vi "CCD.vi"() -> ()   [LabVIEW 2016]
uses:
  <vilib>/userdefined/High Color/IMAQdx.ctl
  <vilib>/UPVI/lvhdf5/file.llb/LVH5F Operation.ctl
  <vilib>/UPVI/lvhdf5/dataset.llb/LVH5D Operation.ctl
  <vilib>/Utility/miscctls.llb/LVRectTypeDef.ctl
  <vilib>/UPVI/lvhdf5/group.llb/H5G_obj_t.ctl
  <vilib>/UPVI/lvhdf5/utility.llb/Select HDF5 Dialog.vi
  <vilib>/UPVI/lvhdf5/utility.llb/Select HDF5 Dialog (Object Only).vi
  <vilib>/UPVI/lvhdf5/dataset.llb/Simple H5Dwrite (Variant).vi
  <vilib>/UPVI/lvhdf5/dataset.llb/Simple H5Dwrite.xnode
  <vilib>/UPVI/lvhdf5/library.llb/HDF5 Ref.ctl
  <vilib>/vision/driver/NI_Vision_Acquisition_Software.lvlib
  <instrlib>/Ocean Optics 2000 4000/Ocean Optics 2000 4000.lvlib
  <vilib>/UPVI/lvhdf5/identifier.llb/Not an HDF5 Refnum Constant.vi
  <vilib>/Utility/error.llb/Error Cluster From Error Code.vi
  <vilib>/UPVI/lvhdf5/dataset.llb/OpenCreateReplace Dataset by Element Type.vi
  <vilib>/UPVI/lvhdf5/dataspace.llb/H5Sselect_hyperslab.vi
  <vilib>/UPVI/lvhdf5/dataset.llb/H5Dwrite (Variant).vi
  <vilib>/UPVI/lvhdf5/dataset.llb/H5Dget_space.vi
  <vilib>/UPVI/lvhdf5/attribute.llb/private/LVH5AwriteWDTAttrs.vi
  <vilib>/UPVI/lvhdf5/dataspace.llb/H5Sclose.vi
  <vilib>/UPVI/lvhdf5/dataset.llb/H5Dclose.vi
  <vilib>/UPVI/lvhdf5/utility.llb/Select HDF5 Dialog (File and Object).vi
panel:
  in  "Tiempo entre muestra (ms)":u32=1000
  in  "Guarda":bool
  out "vy":dbl(slide) scale=-10.0..10.0
  in  "Tiempo de avanze (ms)":u32=100
  in  "Valor final en y":dbl
  in  "Movimiento de spot en y":dbl(slide) scale=-10.0..10.0
  in  "Valor final en  x":dbl
  in  "Paso":dbl=0.01
  out "vx":dbl(slide) scale=-10.0..10.0
  in  "Modo de operación":enum32{"Manual", "Mapeo"}(radio)
  in  "stop":bool
  in  "Movimiento de spot en x":ext(slide) scale=-10.0..10.0
  in  "error in":errorcluster
  out "Guarda datos":bool
  in  "Ruta":path=path "C:/Users/Posgrado/Desktop/Test/Prueba"
  in  "Dataset Path":string="Mapeo"
  in  "No. de muestras":i32=1
  in  "Session In":T1="cam2"
  in  "Enable Strobe (Disabled)":bool
  in  "VISA resource name":refnum<visa-resource-name>="USB0::0x2457::0x1012::NI-VISA-10002::RAW"
  out "Image":T2(plugin-control)
  out "Spectral Waveform":cluster{dbl[], dbl[]}(graph)
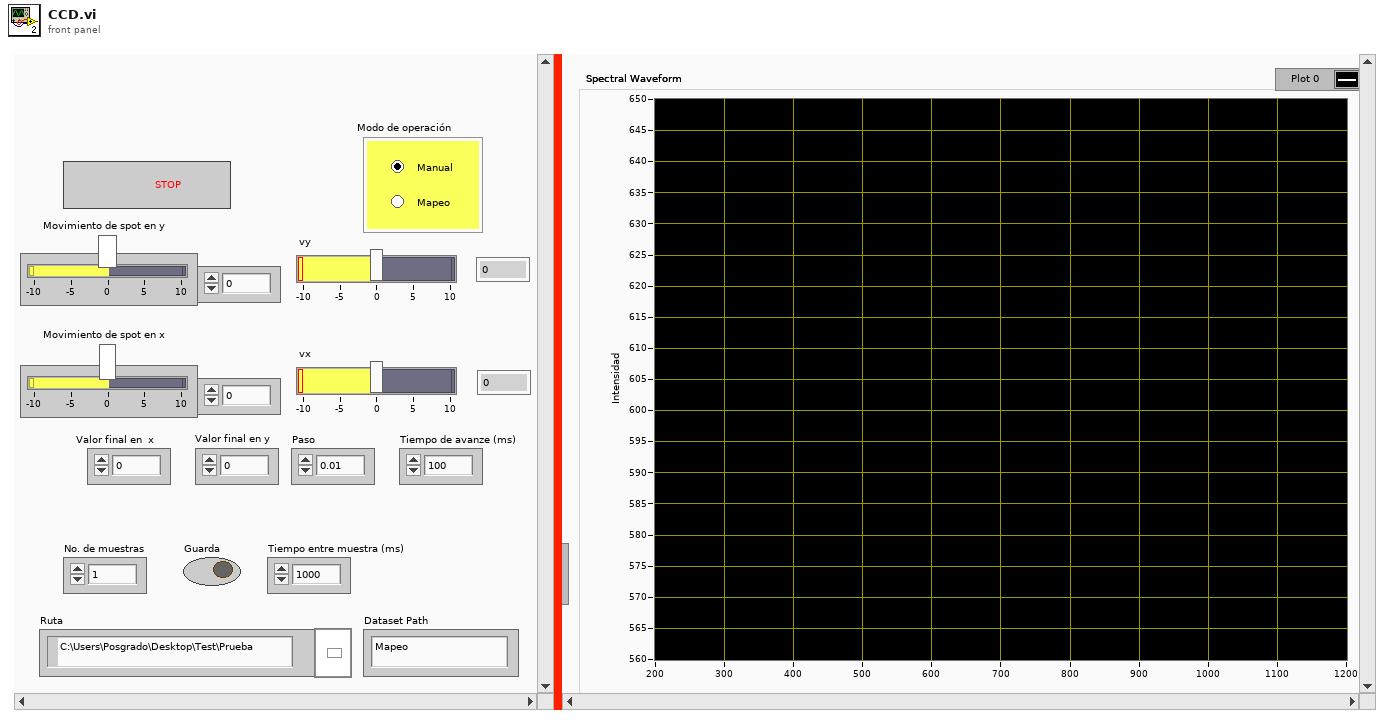
[diagram p1: front panel]
types:
  T1 = typedef "IMAQdx.ctl" = refnum<k21>
  T2 = typedef "IMAQ Image.ctl" = refnum<image>
  T3 = typedef "Image Type" = u32
  T4 = typedef "LVH5D Operation.ctl" = enum16{"open", "replace", "create", "open or create", "create or replace", "create or replace with confirmation"}
  T5 = typedef "LVH5F Operation.ctl" = enum16{"open", "open or create", "create or replace", "create or replace (with confirmation)", "create", "open (read only)"}
  T6 = typedef "LVRectTypeDef.ctl" = cluster{"Left":i16, "Top":i16, "Right":i16, "Bottom":i16}
  T7 = cluster{"Behavior":enum32{"Invalid", "Default", "Floating", "Floating/Auto-Hide", "Modal"}, "Position":T6, "Center":bool, "Title":string}
  T8 = typedef "H5G_obj_t.ctl" = i32
  T9 = cluster{"Object Types (any)":T8[], "Object Pattern":string}
  T10 = typedef "HDF5 Ref.ctl" = refnum<k1>
  T11 = cluster{"Spectrum by Pixel Number":dbl[], "Wavelength (nm)":dbl[]}
  T12 = enum8{"Enabled", "Disabled", "Disabled and Grayed Out"}
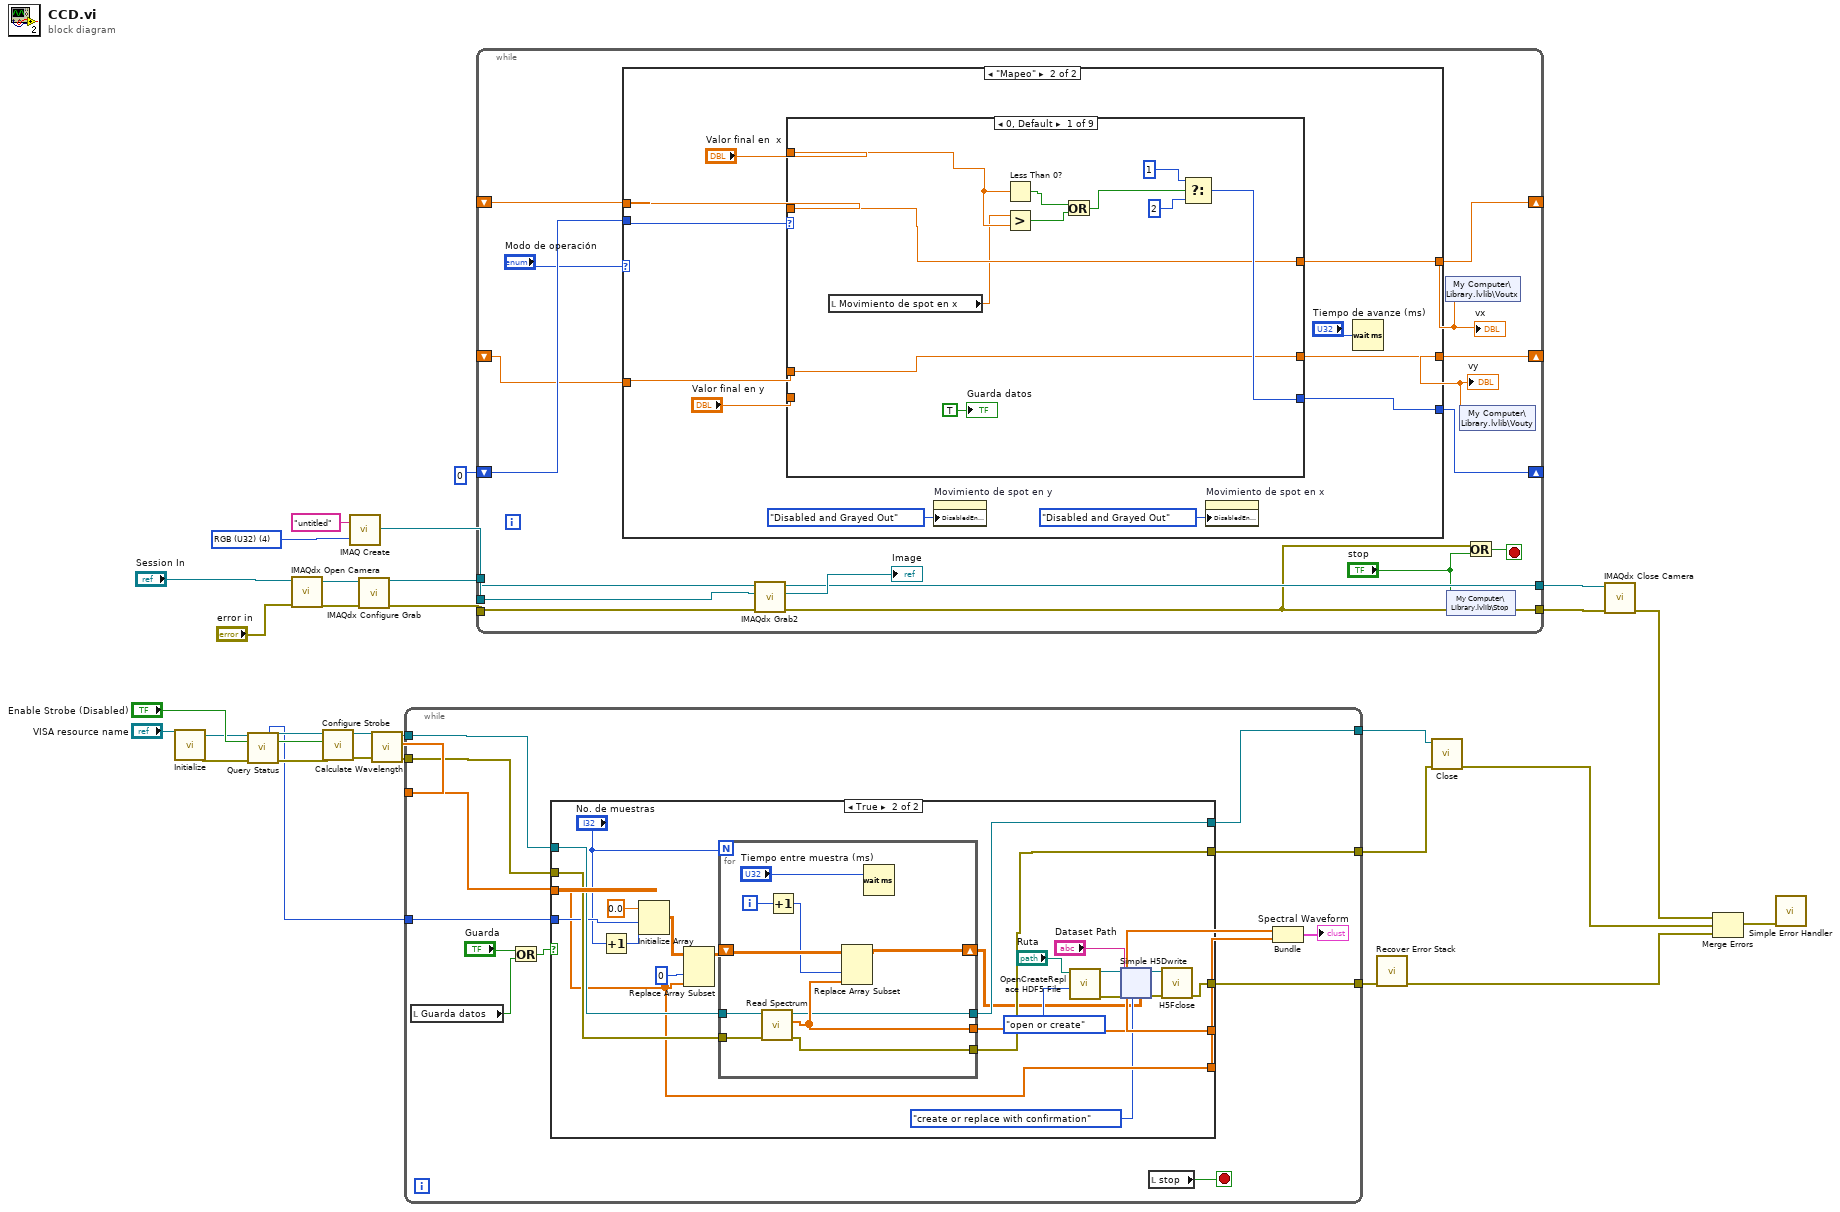
[diagram p0: block diagram]
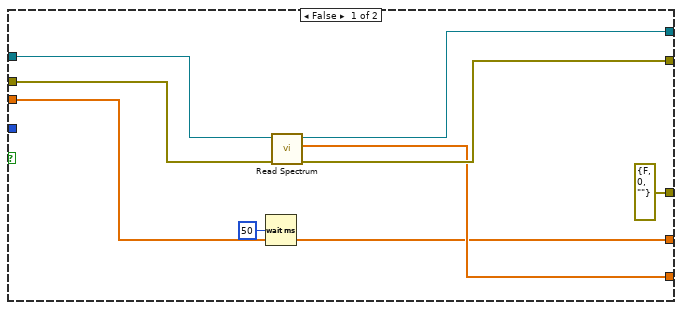
[diagram p2: hidden frame]
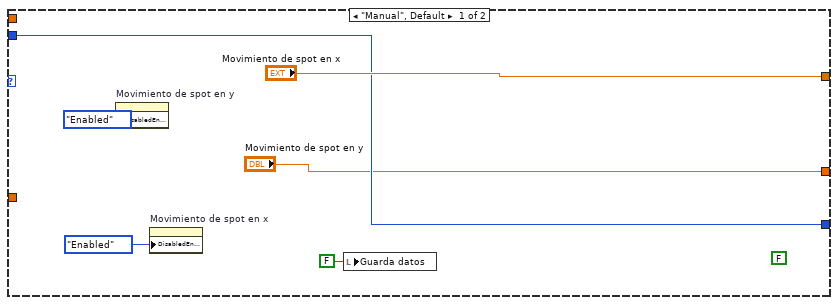
[diagram p3: hidden frame]
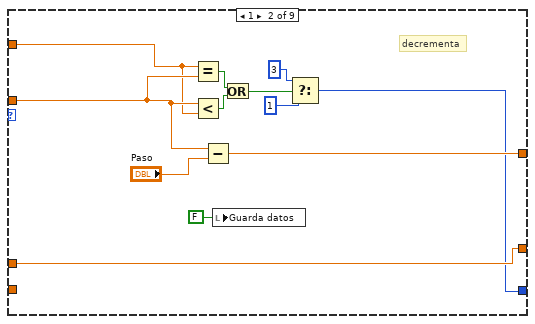
[diagram p4: hidden frame]
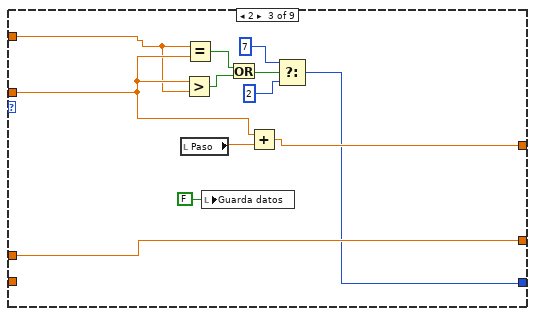
[diagram p5: hidden frame]
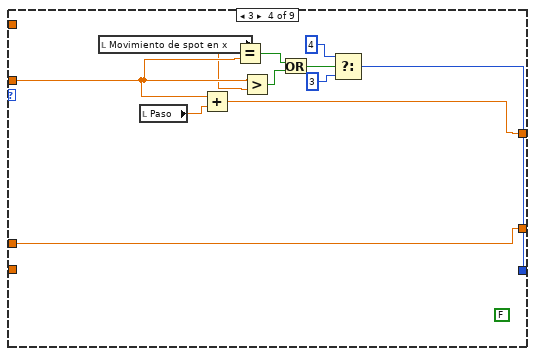
[diagram p6: hidden frame]
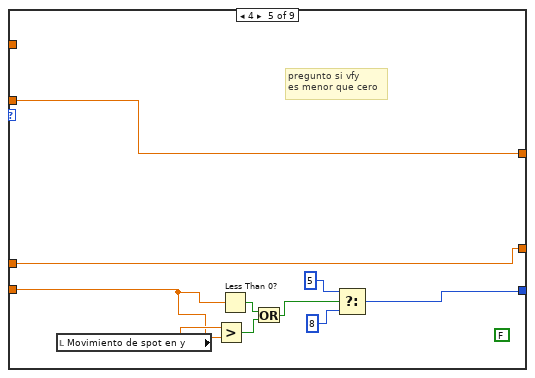
[diagram p7: hidden frame]
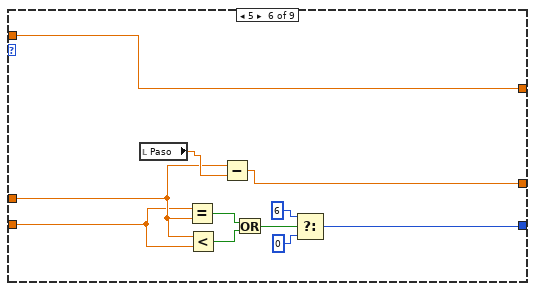
[diagram p8: hidden frame]
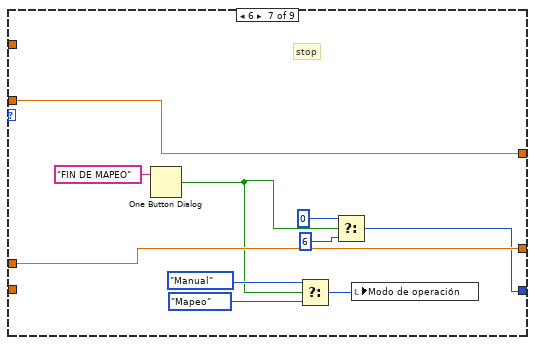
[diagram p9: hidden frame]
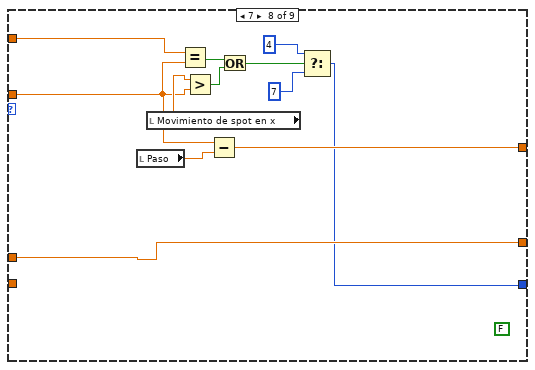
[diagram p10: hidden frame]
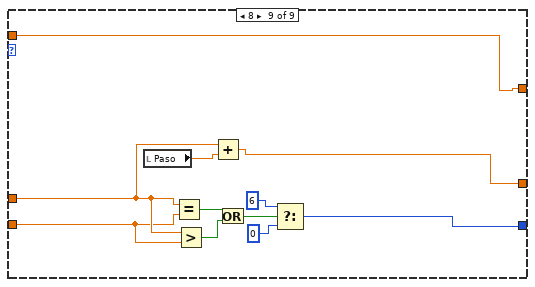
[diagram p11: hidden frame]
diagram:
  w27 = T3 4 items=["Grayscale (U8)", "Grayscale (I16)", "Grayscale (SGL)", "Complex (CSG)", "RGB (U32)", "HSL (U32)", "RGB (U64)", "Grayscale (U16)"] ("Image Type")
  n1 = call <instrlib>:"Initialize.vi"("VISA resource name"="VISA resource name") -> ("error out"=w6:errorcluster, "VISA resource name out"=w7:refnum<visa-resource-name>)  [unwired: 2 in, 7 out]
  n2 = call <instrlib>:"Query Status.vi"("VISA resource name"=w7, "error in (no error)"=w6) -> ("Number of Pixels"=w4:u16, "VISA resource name out"=w8:refnum<visa-resource-name>, "error out"=w5:errorcluster)  [unwired: 11 out]
  n3 = call <vilib>:"IMAQdx Open Camera.vi"("error in"="error in", "Session In"="Session In") -> ("error out"=w29:errorcluster, "Session Out"=w30:T1)  [unwired: 8 in]
  n4 = call <instrlib>:"Configure Strobe.vi"("error in (no error)"=w5, "Enable Strobe (Disabled)"="Enable Strobe (Disabled)", "VISA resource name"=w8) -> ("error out"=w13:errorcluster, "VISA resource name out"=w14:refnum<visa-resource-name>)  [unwired: 7 out]
  n5 = call "IMAQ Create"("Image Name"="untitled", "Image Type"=w27) -> ("New Image"=w22:T2)  [unwired: 3 in, 1 out]
  n6 = call <vilib>:"IMAQdx Configure Grab.vi"("error in"=w29, "Session In"=w30) -> ("error out"=w23:errorcluster, "Session Out"=w24:T1)  [unwired: 8 in]
  n7 = call <instrlib>:"Calculate Wavelength.vi"("error in (no error)"=w13, "VISA resource name"=w14) -> ("error out"=w15:errorcluster, "Wavelength (nm)"=w17:dbl[], "VISA resource name out"=w16:refnum<visa-resource-name>)  [unwired: 1 in, 6 out]
  n8 = while {
    tunnel: w17 -> [w42]
    tunnel: w16 -> [w44]
    tunnel: w15 -> [w43]
    tunnel: w4 -> [w41]
    tunnel: [w40] -> w3
    tunnel: [w39] -> w2
    tunnel: [w35] -> w1
    stop <- w45 stop-if-true
    n9 = local read "Guarda datos"() -> (w32:bool)
    n10 = Or(x="Guarda", y=w32) -> (x .or. y?=w34:bool)
    n11 = case shown="True" w34 {
      tunnel: w44 -> [w53 w76]
      tunnel: w43 -> [w52 w75]
      tunnel: w42 -> [w47 w66]
      tunnel: w41 -> [_ w71]
      tunnel: [w50 w65] -> w40
      tunnel: [w49 w64] -> w39
      tunnel: [w48 w66] -> w37
      tunnel: [w47 w67] -> w36
      tunnel: [errorcluster {"status"=FALSE, "code"=0, "source"=""} ("error out") w54] -> w35
      frame False {
        n12 = Wait (ms)(milliseconds to wait=u32 50) -> ()  [unwired: 1 out]
        n13 = call <instrlib>:"Read Spectrum.vi"("error in (no error)"=w52, "VISA resource name"=w53) -> ("error out"=w49:errorcluster, "Spectrum by Pixel Number"=w48:dbl[], "VISA resource name out"=w50:refnum<visa-resource-name>)  [unwired: 6 in, 1 out]
      }
      frame True {
        n14 = Increment(x="No. de muestras") -> (x+1=w69:i32)
        n15 = Initialize Array(0.0 ("element"), w71, w69) -> (w73:dbl[][])
        n16 = Replace Array Subset(array=w73, new element=w66, index (col)=0) -> (w68:dbl[][])  [unwired: 1 in]
        n17 = for {
          N: "No. de muestras" -> [_]
          tunnel: w76 -> [w288]
          tunnel: w75 -> [w287]
          shift-right: [w285] -> w55
          shift-left: w68 -> [w286]
          tunnel: [w282] -> w67
          tunnel: [w281] -> w65
          tunnel: [w280] -> w64
          i -> [w284]
          n18 = call <instrlib>:"Read Spectrum.vi"("error in (no error)"=w287, "VISA resource name"=w288) -> ("error out"=w280:errorcluster, "Spectrum by Pixel Number"=w282:dbl[], "VISA resource name out"=w281:refnum<visa-resource-name>)  [unwired: 6 in, 1 out]
          n19 = Increment(x=w284) -> (x+1=w283:i32)
          n20 = Replace Array Subset(array=w286, new element=w282, index (col)=w283) -> (w285:dbl[][])  [unwired: 1 in]
          n21 = Wait (ms)(milliseconds to wait="Tiempo entre muestra (ms)") -> ()  [unwired: 1 out]
        }
        n22 = call <vilib>:"OpenCreateReplace HDF5 File.vi"("function (open or create)"=LVH5F_Operation."open or create", "path"="Ruta") -> ("error out"=w61:errorcluster, "HDF5 Ref out"=w60:T10)  [unwired: 6 in]
        n23 = xnode "Simple H5Dwrite"("Dataset Path"="Dataset Path", "error in (no error)"=w61, "operation (open or create)"=LVH5D_Operation."create or replace with confirmation", "HDF5 Path or Ref"=w60, "Data"=w55) -> ("HDF5 Ref out"=w57:T10, "error out"=w58:errorcluster)  [unwired: 3 in, 1 out]
        n24 = call <vilib>:"H5Fclose.vi"("error in (no error)"=w58, "HDF5 Ref"=w57) -> ("error out"=w54:errorcluster)  [unwired: 7 in]
      }
    }
    n25 = local read "stop"() -> (w45:bool)
    n26 = Bundle("Spectrum by Pixel Number"=w36, "Wavelength (nm)"=w37) -> (→"Spectral Waveform":T11)  [unwired: 1 out]
  }
  n27 = while {
    shift-right: [w298] -> _
    shift-left: _ -> [w304]
    shift-right: [w302] -> _
    shift-left: 0 -> [w303]
    shift-right: [w299] -> _
    shift-left: _ -> [w301]
    tunnel: w24 -> [w295]
    tunnel: w23 -> [w294]
    tunnel: w22 -> [w293]
    tunnel: [w292] -> w21
    tunnel: [w289] -> w20
    stop <- w300 stop-if-true
    n28 = case shown="\"Mapeo\"" "Modo de operación" {
      tunnel: ["Movimiento de spot en x" w314] -> w298
      tunnel: w304 -> [_ w321]
      tunnel: w303 -> [w309 w311]
      tunnel: [w309 w316] -> w302
      tunnel: ["Movimiento de spot en y" w315] -> w299
      tunnel: w301 -> [_ w319]
      frame "Manual", Default {
        (unwired) FALSE ("true")
        n29 = property on="Movimiento de spot en y" class="Slide (strict)"("DisabledEnum"=T12."Enabled" ("Disabled")) -> ()  [unwired: 2 in, 2 out]
        n30 = property on="Movimiento de spot en x" class="Slide (strict)"("DisabledEnum"=T12."Enabled" ("Disabled")) -> ()  [unwired: 2 in, 2 out]
        n31 = local write "Guarda datos"(FALSE ("Guarda datos")) -> ()
      }
      frame "Mapeo" {
        n32 = case shown="0, Default" w311 {
          tunnel: w321 -> [w328 w338 w353 w365 w377 w388 w398 w399 w421]
          tunnel: "Valor final en  x" -> [w327 w337 w352 _ _ _ _ w406 _]
          tunnel: w319 -> [w329 w344 w356 w357 w376 w380 w397 w410 w413]
          tunnel: "Valor final en y" -> [_ _ _ _ w371 w379 _ _ w412]
          tunnel: [w331 w339 w348 w359 w374 w385 w390 w407 w415] -> w316
          tunnel: [w329 w344 w356 w357 w376 w383 w397 w410 w419] -> w315
          tunnel: [w328 w342 w354 w366 w377 w388 w398 w408 w421] -> w314
          frame 0, Default {
            n33 = local read "Movimiento de spot en x"() -> (w323:ext)
            n34 = Less Than 0?(x=w327) -> (x < 0?=w325:bool)
            n35 = Greater?(x=w323, y=w327) -> (0:w326:bool)
            n36 = Or(x=w325, y=w326) -> (x .or. y?=w324:bool)
            n37 = Select(t=1, s=w324, f=2) -> (s? t:f=w331:i32)
            "Guarda datos" <- TRUE ("Guarda datos")
          }
          frame 1 {
            # "decrementa"
            n38 = Equal?(x=w337, y=w338) -> (x = y?=w335:bool)
            n39 = Less?(x=w338, y=w337) -> (x < y?=w336:bool)
            n40 = Subtract(x=w338, y="Paso") -> (x-y=w342:ext)
            n41 = local write "Guarda datos"(FALSE ("Guarda datos")) -> ()
            n42 = Or(x=w335, y=w336) -> (x .or. y?=w334:bool)
            n43 = Select(t=3, s=w334, f=1) -> (s? t:f=w339:i32)
          }
          frame 2 {
            n44 = local read "Paso"() -> (w355:dbl)
            n45 = Greater?(x=w353, y=w352) -> (0:w351:bool)
            n46 = Equal?(x=w352, y=w353) -> (x = y?=w350:bool)
            n47 = local write "Guarda datos"(FALSE ("Guarda datos")) -> ()
            n48 = Or(x=w350, y=w351) -> (x .or. y?=w349:bool)
            n49 = Add(x=w353, y=w355) -> (x+y=w354:ext)
            n50 = Select(t=7, s=w349, f=2) -> (s? t:f=w348:i32)
          }
          frame 3 {
            (unwired) FALSE ("true")
            n51 = local read "Movimiento de spot en x"() -> (w364:ext)
            n52 = local read "Paso"() -> (w367:dbl)
            n53 = Add(x=w365, y=w367) -> (x+y=w366:ext)
            n54 = Equal?(x=w364, y=w365) -> (x = y?=w362:bool)
            n55 = Greater?(x=w365, y=w364) -> (0:w363:bool)
            n56 = Or(x=w362, y=w363) -> (x .or. y?=w361:bool)
            n57 = Select(t=4, s=w361, f=3) -> (s? t:f=w359:i32)
          }
          frame 4 {
            (unwired) FALSE ("true")
            # "pregunto si vfy\nes menor que cero"
            n58 = local read "Movimiento de spot en y"() -> (w372:dbl)
            n59 = Greater?(x=w372, y=w371) -> (0:w369:bool)
            n60 = Less Than 0?(x=w371) -> (x < 0?=w370:bool)
            n61 = Or(x=w370, y=w369) -> (x .or. y?=w368:bool)
            n62 = Select(t=5, s=w368, f=8) -> (s? t:f=w374:i32)
          }
          frame 5 {
            n63 = local read "Paso"() -> (w384:dbl)
            n64 = Equal?(x=w379, y=w380) -> (x = y?=w381:bool)
            n65 = Less?(x=w380, y=w379) -> (x < y?=w378:bool)
            n66 = Subtract(x=w380, y=w384) -> (x-y=w383:dbl)
            n67 = Or(x=w381, y=w378) -> (x .or. y?=w382:bool)
            n68 = Select(t=6, s=w382, f=0) -> (s? t:f=w385:i32)
          }
          frame 6 {
            # "stop"
            n69 = One Button Dialog(message="FIN DE MAPEO") -> (true=w392:bool)  [unwired: 1 in]
            n70 = Select(t=enum32{"Manual", "Mapeo"}."Manual" ("Modo de operación"), s=w392, f=enum32{"Manual", "Mapeo"}."Mapeo") -> (s? t:f=w394:enum32{"Manual", "Mapeo"})
            n71 = Select(t=0, s=w392, f=6) -> (s? t:f=w390:i32)
            n72 = local write "Modo de operación"(w394) -> ()
          }
          frame 7 {
            (unwired) FALSE ("true")
            n73 = local read "Paso"() -> (w409:dbl)
            n74 = local read "Movimiento de spot en x"() -> (w400:ext)
            n75 = Equal?(x=w406, y=w399) -> (x = y?=w405:bool)
            n76 = Greater?(x=w400, y=w399) -> (0:w401:bool)
            n77 = Subtract(x=w399, y=w409) -> (x-y=w408:ext)
            n78 = Or(x=w405, y=w401) -> (x .or. y?=w404:bool)
            n79 = Select(t=4, s=w404, f=7) -> (s? t:f=w407:i32)
          }
          frame 8 {
            n80 = local read "Paso"() -> (w420:dbl)
            n81 = Equal?(x=w413, y=w412) -> (x = y?=w418:bool)
            n82 = Greater?(x=w413, y=w412) -> (0:w414:bool)
            n83 = Add(x=w413, y=w420) -> (x+y=w419:dbl)
            n84 = Or(x=w418, y=w414) -> (x .or. y?=w417:bool)
            n85 = Select(t=6, s=w417, f=0) -> (s? t:f=w415:i32)
          }
        }
        n86 = property on="Movimiento de spot en y" class="Slide (strict)"("DisabledEnum"=T12."Disabled and Grayed Out" ("Disabled")) -> ()  [unwired: 2 in, 2 out]
        n87 = property on="Movimiento de spot en x" class="Slide (strict)"("DisabledEnum"=T12."Disabled and Grayed Out" ("Disabled")) -> ()  [unwired: 2 in, 2 out]
        n88 = Wait (ms)(milliseconds to wait="Tiempo de avanze (ms)") -> ()  [unwired: 1 out]
      }
    }
    "vx" <- w298
    "vy" <- w299
    n89 = call <vilib>:"IMAQdx Grab2.vi"("error in"=w294, "Image In"=w293, "Session In"=w295) -> ("error out"=w290:errorcluster, "Image Out"=→"Image":T2, "Session Out"=w292:T1)  [unwired: 5 in, 1 out]
    n90 = shared-variable "My Computer\\Library.lvlib\\Voutx"(w298) -> ()  [unwired: 1 in, 1 out]
    n91 = shared-variable "My Computer\\Library.lvlib\\Stop"("stop", error in=w290) -> (error out=w289:errorcluster)
    n92 = shared-variable "My Computer\\Library.lvlib\\Vouty"(w299) -> ()  [unwired: 1 in, 1 out]
    n93 = Or(x=w290, y="stop") -> (x .or. y?=w300:bool)
  }
  n94 = call <vilib>:"Recover Error Stack.vi"("error in (no error)"=w1) -> ("error out"=w10:errorcluster)  [unwired: 5 in, 3 out]
  n95 = call <instrlib>:"Close.vi"("error in (no error)"=w2, "VISA resource name"=w3) -> ("error out"=w9:errorcluster)  [unwired: 9 out]
  n96 = call <vilib>:"IMAQdx Close Camera.vi"("error in"=w20, "Session In"=w21) -> ("error out"=w11:errorcluster)  [unwired: 9 in]
  n97 = Merge Errors(w11, w9, w10) -> (w12:errorcluster)
  n98 = call <vilib>:"Simple Error Handler.vi"("error in (no error)"=w12) -> ()  [unwired: 4 in, 5 out]
